vi "setSetpoint.vi"(8 "error in (no error)":errorcluster, 9 "Force Setpoint":dbl[unit], 10 "ILC in":refnum<class "ILC.lvclass">, 11 "IActuator in":refnum<class "IActuator.lvclass">) -> (0 "error out":errorcluster, 2 "ILC out":refnum<class "ILC.lvclass">, 3 "IActuator out":refnum<class "IActuator.lvclass">)   [LabVIEW 2015, in "IActuator.lvclass"]
uses:
  IActuator.lvclass
  <userlib>/Common/ILC/ILC/ILC.lvclass
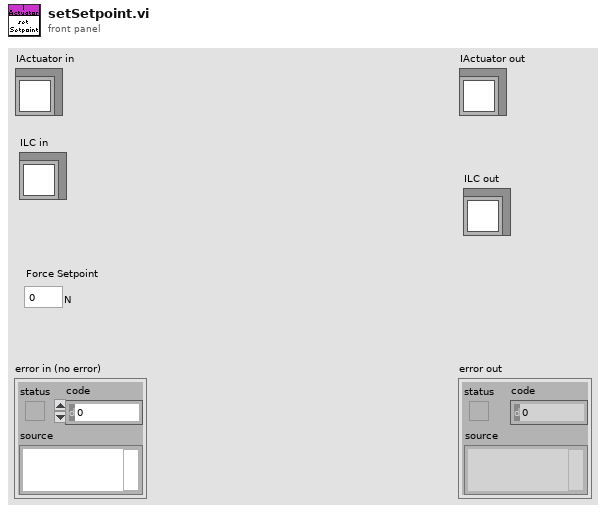
[diagram p1: front panel]
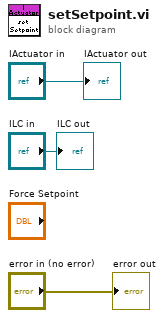
[diagram p0: block diagram]
diagram:
  "error out" <- "error in (no error)"
  "IActuator out" <- "IActuator in"
  "ILC out" <- "ILC in"
